vi "DG_Setup.vi"(7 "Path":path=path "C:/G0X/Data", 8 "error in (no error)":errorcluster, 11 "Select Product":i32(ring) items=["SRS_DG135"=1, "BME_DP01"=2, "BME_G02V3"=3, "BME_SG02V4"=4, "BME_G04"=5, "BME_G02V1"=6, "BME_G02V2"=7, "BME_SG02V1"=8, "BME_SG02V2"=9, "BME_SG02V3"=10, "BME_G03V1"=11, "BME_G03V2"=12, "BME_SG02V5"=13, "BME_G03V3"=14, "BME_G03V4"=15, "BME_SG02V6"=16, "BME_G03V5"=17, "BME_G05V1"=18, "BME_G05V2"=19, "BME_G05V3"=20, "BME_SG02V7"=21, "BME_SG02P1"=31, "BME_G03P1"=32, "BME_G05P1"=33, "BME_SG02P2"=34, "BME_G03P2"=35, "BME_SG02P3"=36, "BME_SG05P1"=37, "BME_G05P2"=38, "BME_SG05P2"=39, "BME_G05P3"=40, "BME_SG02P4"=41, "BME_SG02P5"=42, "BME_SG05P3"=43, "BME_SG08P1"=44]) -> (0 "error out":errorcluster, 3 "DG Number":i32, 5 "Generator Info":T1(array[cluster]) {"DG Product" items=["SRS_DG135"=1, "BME_DP01"=2, "BME_G02V3"=3, "BME_SG02V4"=4, "BME_G04"=5, "BME_G02V1"=6, "BME_G02V2"=7, "BME_SG02V1"=8, "BME_SG02V2"=9, "BME_SG02V3"=10, "BME_G03V1"=11, "BME_G03V2"=12, "BME_SG02V5"=13, "BME_G03V3"=14, "BME_G03V4"=15, "BME_SG02V6"=16, "BME_G03V5"=17, "BME_G05V1"=18, "BME_G05V2"=19, "BME_G05V3"=20, "BME_SG02V7"=21, "BME_SG02P1"=31, "BME_G03P1"=32, "BME_G05P1"=33, "BME_SG02P2"=34, "BME_G03P2"=35, "BME_SG02P3"=36, "BME_SG05P1"=37, "BME_G05P2"=38, "BME_SG05P2"=39, "BME_G05P3"=40, "BME_SG02P4"=41, "BME_SG02P5"=42, "BME_SG05P3"=43, "BME_SG08P1"=44]})   [LabVIEW 2009, in "POLARIS BME DG.lvlib"]
uses:
  POLARIS BME DG.lvlib
panel:
  # "NOTICE -- YOU MUST LEAVE THIS NOTICE IN PLACE.  PER THE TERMS OF THE LICENSE BELOW, YOU MAY SUBLICENSE THIS SOFTWARE \nIN ANY WAY THAT DOES NOT CONFLICT WITH THIS LICENSE.\n\n### BSD License (http://www.opensource.org/licenses/bsd-license.php) Begin ###\n \nCopyright (c) 2011, Applied Energetics, http://www.appliedenergetics.com,\n                               Richard Schwerdtfeger, <rschwerdtfeger@appliedenergetics.com>\n\nAll rights reserved.\n\nRedistribution and use in source and binary forms, with or without modification, are permitted provided that the \nfollowing conditions are met:\n\n    * Redistributions of source code must retain the above copyright notice, this list of conditions and the following disclaimer.\n    * Redistributions in binary form must reproduce the above copyright notice, this list of conditions and the following disclaimer \n       in the documentation and/or other materials provided with the distribution.\n    * Neither the name of Richard Schwerdtfeger, Applied Energetics, Inc., nor the names of its contributors may be used to \n       endorse or promote products derived from this software without specific prior written permission.\n\nTHIS SOFTWARE IS PROVIDED BY THE COPYRIGHT HOLDERS AND CONTRIBUTORS \"AS IS\" AND ANY EXPRESS OR IMPLIED WARRANTIES, \nINCLUDING, BUT NOT LIMITED TO, THE IMPLIED WARRANTIES OF MERCHANTABILITY AND FITNESS FOR A PARTICULAR PURPOSE ARE \nDISCLAIMED. IN NO EVENT SHALL THE COPYRIGHT OWNER OR CONTRIBUTORS BE LIABLE FOR ANY DIRECT, INDIRECT, INCIDENTAL,\n SPECIAL, EXEMPLARY, OR CONSEQUENTIAL DAMAGES (INCLUDING, BUT NOT LIMITED TO, PROCUREMENT OF SUBSTITUTE GOODS OR \nSERVICES; LOSS OF USE, DATA, OR PROFITS; OR BUSINESS INTERRUPTION) HOWEVER CAUSED AND ON ANY THEORY OF LIABILITY, \nWHETHER IN CONTRACT, STRICT LIABILITY, OR TORT (INCLUDING NEGLIGENCE OR OTHERWISE) ARISING IN ANY WAY OUT OF THE USE \nOF THIS SOFTWARE, EVEN IF ADVISED OF THE POSSIBILITY OF SUCH DAMAGE.\n\n### BSD License End ###"
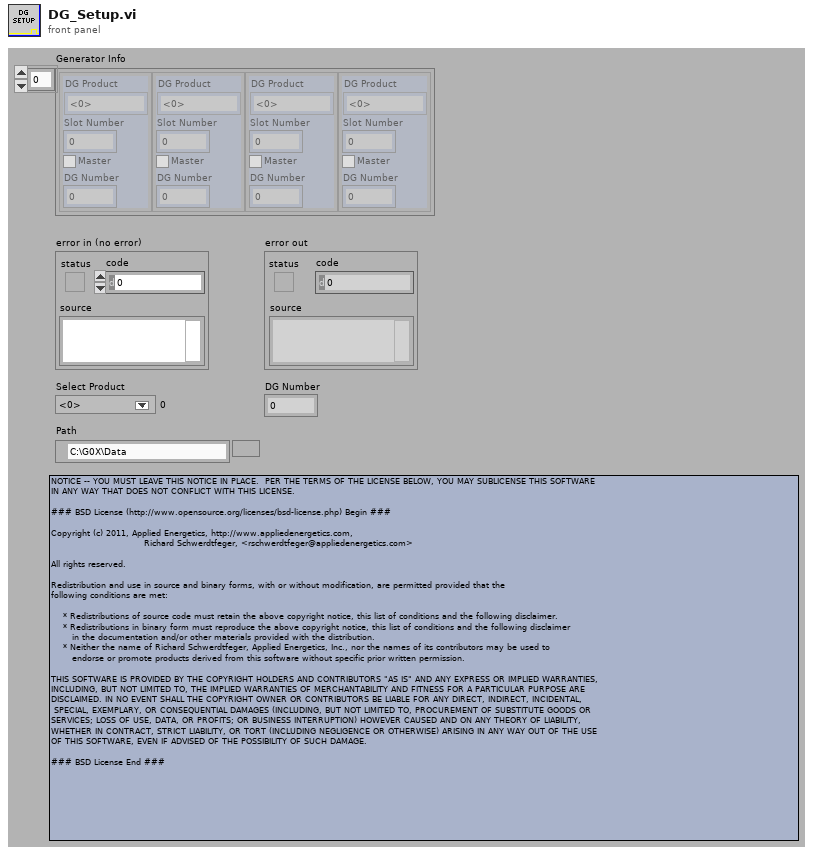
[diagram p1: front panel]
types:
  T1 = cluster{"DG Product":i32, "Slot Number":i32, "Master":bool, "DG Number":i32}[]
  T2 = cluster{"DG Product":i32, "Slot Number":i32, "Master":bool, "DG Number":i32}
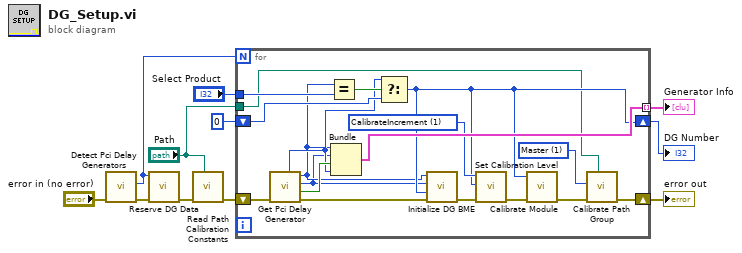
[diagram p0: block diagram]
diagram:
  n1 = call "Detect Pci Delay Generators.vi"("error in (no error)"="error in (no error)") -> ("error out"=w5:errorcluster, "Number of Generators"=w3:i32)  [unwired: 9 out]
  n2 = call "Reserve DG Data.vi"("error in (no error)"=w5, "Number Of Delay Generators"=w3) -> ("error out"=w4:errorcluster)  [unwired: 9 out]
  n3 = call "Read Path Calibration Constants.vi"("Path"="Path", "error in (no error)"=w4) -> ("error out"=w6:errorcluster)  [unwired: 9 out]
  n4 = for {
    N: w3 -> [_]
    shift-right: [w16] -> w2
    shift-left: w6 -> [w29]
    tunnel: [w27] -> w10 mode=indexing
    shift-right: [w15] -> w8
    shift-left: 0 ("DG Number") -> [w26]
    tunnel: "Select Product" -> [w25]
    tunnel: "Path" -> [w14]
    w21 = 1 items=["Master"=1, "Slave"=2] ("Module")
    w20 = u32 1 items=["None", "CalibrateIncrement", "CalibrateOffset"] ("CalibrationLevel")
    n5 = call "Get Pci Delay Generator.vi"("error in (no error)"=w29) -> ("error out"=w18:errorcluster, "Master"=w28:bool, "Slot Number"=w12:i32, "DG Product"=w13:i32, "DG Number"=w23:i32)  [unwired: 6 out]
    n6 = Equal?(x=w13, y=w25) -> (x = y?=w24:bool)
    n7 = Bundle("DG Product"=w13, "Slot Number"=w12, "Master"=w28, "DG Number"=w23) -> (w27:T2)  [unwired: 1 out]
    n8 = Select(t=w23, s=w24, f=w26) -> (s? t:f=w15:i32)
    n9 = call "Initialize DG BME.vi"("error in (no error)"=w18, "DG Number"=w15, "Slot Number"=w12, "DG Product"=w13) -> ("error out"=w22:errorcluster)  [unwired: 7 out]
    n10 = call "Set Calibration Level.vi"("error in (no error)"=w22, "DG Number"=w15, "CalibrationLevel"=w20) -> ("error out"=w19:errorcluster)  [unwired: 8 out]
    n11 = call "Calibrate Module.vi"("error in (no error)"=w19, "DG_Number"=w15) -> ("error out"=w17:errorcluster)  [unwired: 9 out]
    n12 = call "Calibrate Path Group.vi"("Path"=w14, "error in (no error)"=w17, "Module"=w21) -> ("error out"=w16:errorcluster)  [unwired: 8 out]
  }
  "error out" <- w2
  "Generator Info" <- w10
  "DG Number" <- w8
